vi "Check_EnFlo_Arm.vi"() -> ()   [LabVIEW 2010]
uses:
  Gen Trav/Trav_mode.ctl
  ADAM Serial/Instrument drivers/Traverses/~subVIs/DriveConfigGlobal.vi
panel:
  out "Position Output XYZ":dbl[](array[numeric]) format="%.2f"
  in  "Mode":T1(ring)
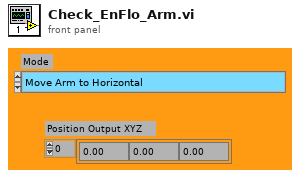
[diagram p1: front panel]
types:
  T1 = enum16{"Move Arm to Horizontal", "Teach Traverse That Arm is Level"}
  T2 = typedef "Trav_mode.ctl" = enum16{"Move traverse", "Read traverse position", "Teach Position"}
  T3 = enum16{"Load setup from excel file", "Save setup to excel file"}
  T4 = typedef "AxisConfigCluster.ctl" = cluster{"Channel Properties":T5, "Static Drive Configuration":T6}
  T5 = typedef "DriveProperties.ctl" = cluster{"Channel Name":string, "Vel. Default":dbl, "Acc. Default":dbl, "Vel. Max":dbl, "Vel. Min":dbl, "Acc. Max":dbl, "Acc. Min":dbl, "Pulses/unit":dbl, "Address":u8, "Pulse Offset":i32, "Pos Tolerance":dbl, "Pulses/rev":dbl, "Backlash/Eng units":dbl, "Current Pos":dbl, "Ch Status":enum16{"Active", "Offline", "Simulate"}, "Port Name":string, "Axis Transform mode":string, "Metadata Ch Name":string, "Type":string}
  T6 = typedef "DriveStaticConfig.ctl" = cluster{"Correction Gain % (CG)":u16, "Dead Band (DB)":i32, "Dead Band Window (DW)":i32, "Encoder Resolution (ER)":i32, "Step Mode  (FSB)":u16, "Position Maintenance (FSC)":u16, "Stop on Stall (FSD)":u16, "Activate OP1 on stall (FSE)":u16, "Stop on Trigger 3 (FSF)":u16, "OP2 in Deadband (FSG)":u16, "Stall Detect (FSH)":u16, "Limit Disable (LD)":u16, "Motor Resolution (MR)":enum16{"200", "400", "1000", "2000", "4000", "5000", "10000", "12800", "18000", "20000", "21600", "25000", "25400", "25600", "36000", "50000", "278528", "425984", "507904", "614400", "655360", "819200", "1024000"}, "Limit Switch Sense (OSA)":u16, "Home Position (OSB)":u16, "Home Switch Sense (OSC)":u16, "Encoder Z for Home (OSD)":u16, "Reference edge of Home (OSH)":u16, "RS232 Echo Control (SSA)":u16, "Buffer at Limit (SSG)":u16, "Buffer at Stop (SSH)":u16, "Indexer Mode  (FSA)":u16, "Type":string, "ConfigString":string, "De Power Motor":enum16{"TRUE", "FALSE"}}
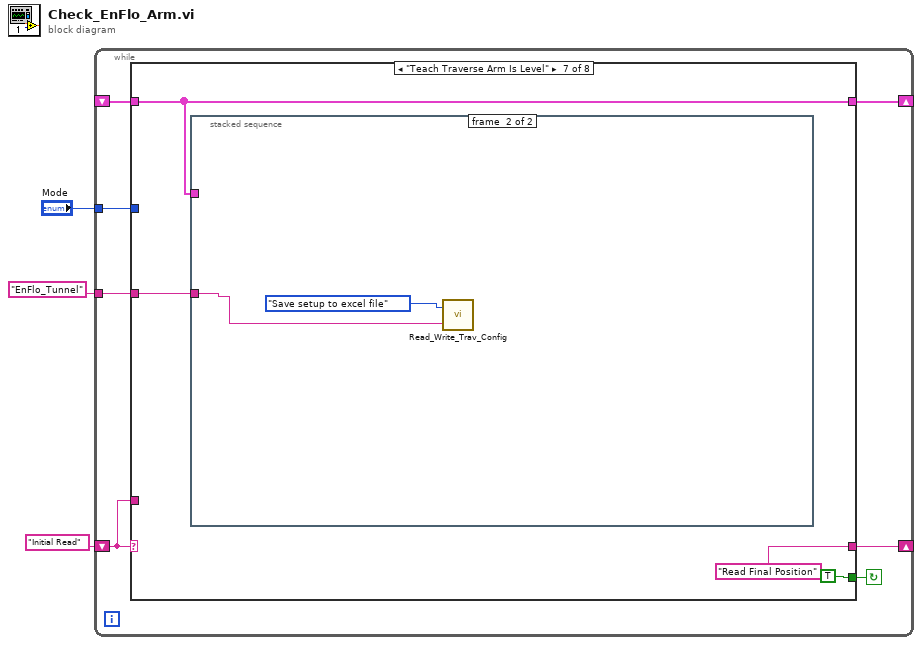
[diagram p0: block diagram]
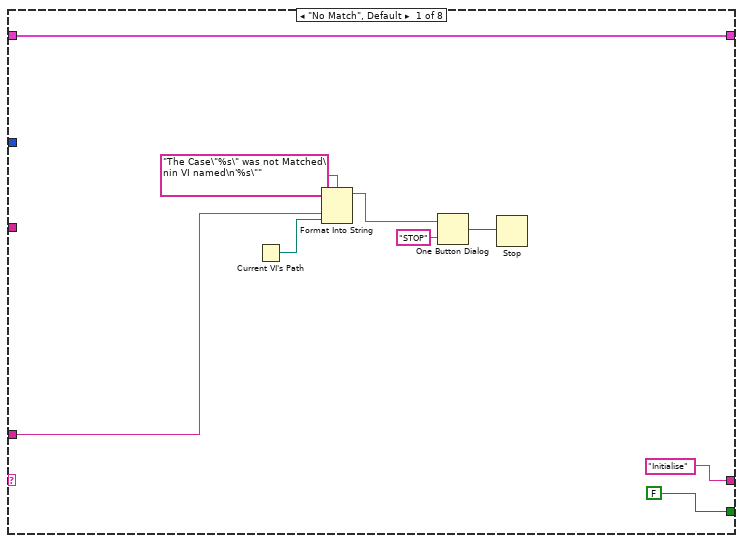
[diagram p2: hidden frame]
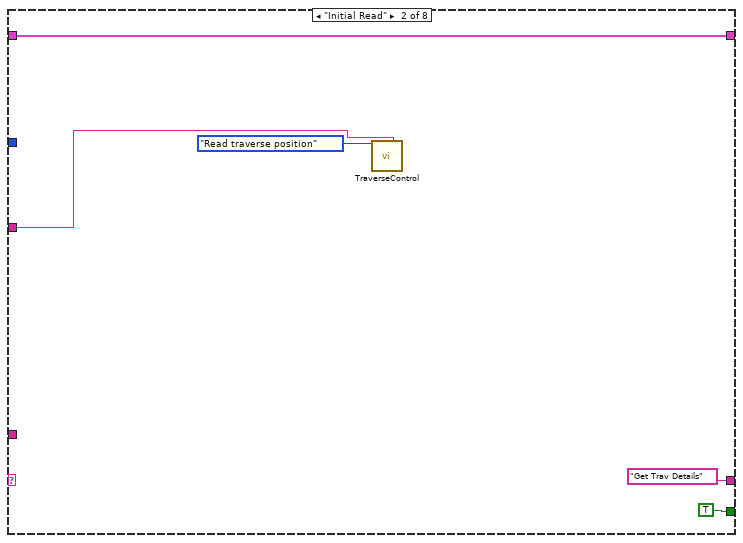
[diagram p3: hidden frame]
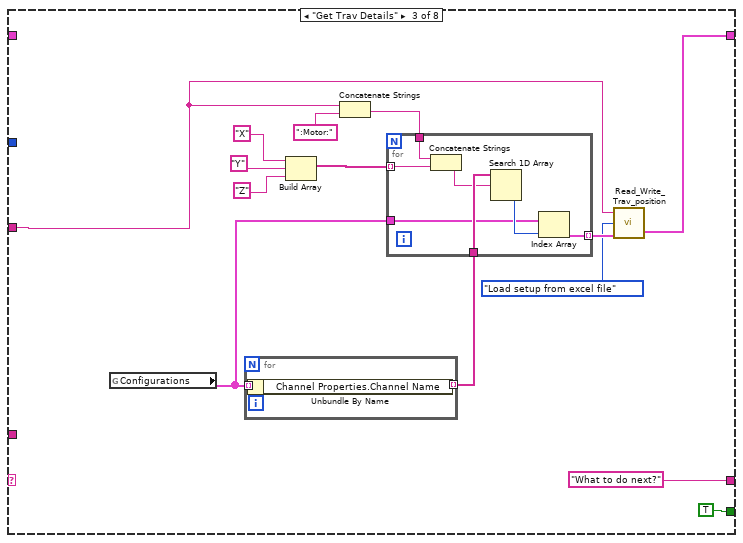
[diagram p4: hidden frame]
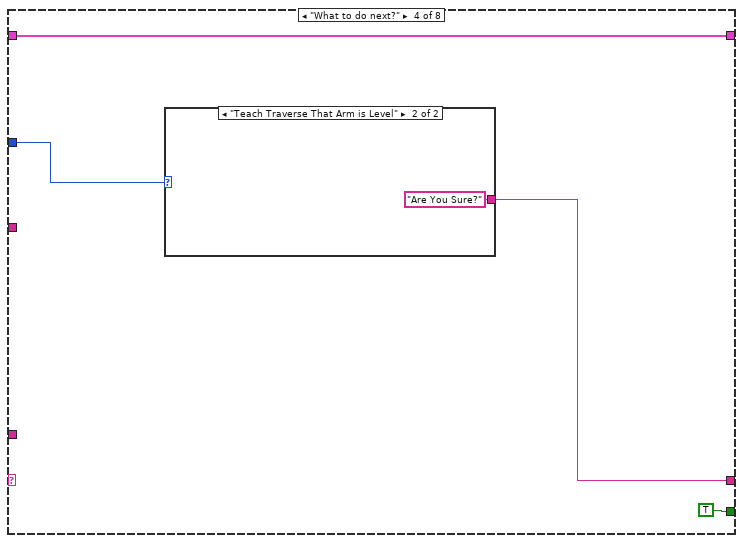
[diagram p5: hidden frame]
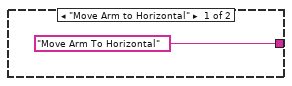
[diagram p6: hidden frame]
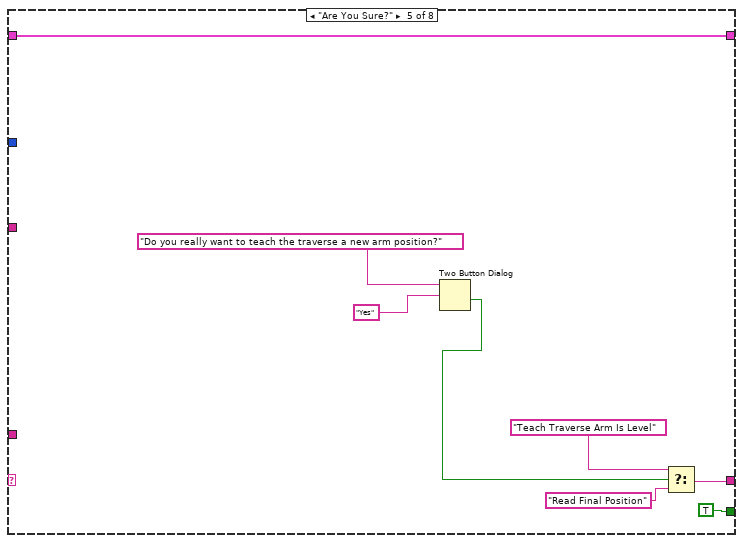
[diagram p7: hidden frame]
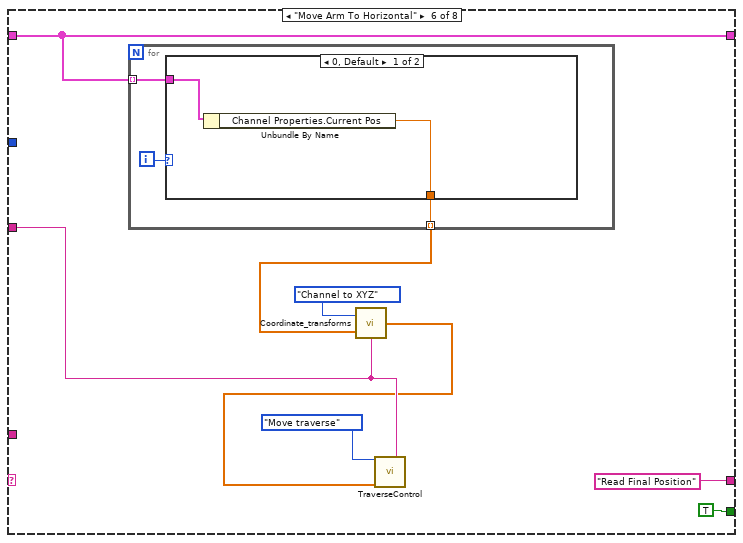
[diagram p8: hidden frame]
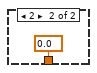
[diagram p9: hidden frame]
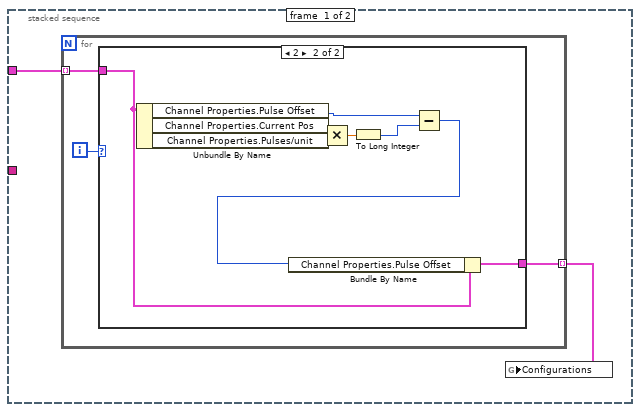
[diagram p10: hidden frame]
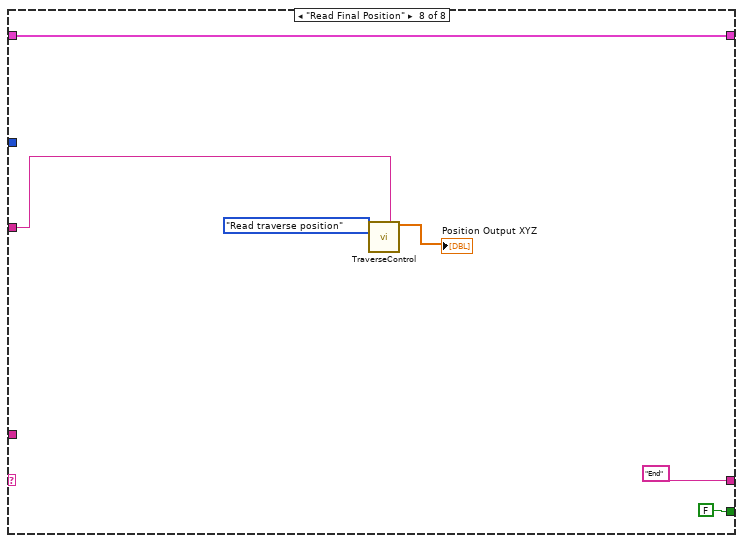
[diagram p12: hidden frame]
diagram:
  n1 = while {
    tunnel: "Mode" -> [w4]
    shift-left: _ -> [w5]
    shift-right: [w6] -> _
    tunnel: "EnFlo_Tunnel" ("Traverse Name") -> [w7]
    shift-left: "Initial Read" -> [w8]
    shift-right: [w9] -> _
    stop <- w10 continue-if-true
    n2 = case shown="\"Teach Traverse Arm Is Level\"" w8 {
      tunnel: [FALSE TRUE TRUE TRUE TRUE TRUE TRUE FALSE] -> w10
      tunnel: ["Initialise" "Get Trav Details" "What to do next?" w49 w55 "Read Final Position" "Read Final Position" "End"] -> w9
      tunnel: w8 -> [w14 _ _ _ _ _ _ _]
      tunnel: w7 -> [_ w20 w26 _ _ w64 w76 w98]
      tunnel: [w11 w21 w25 w48 w60 w67 w77 w97] -> w6
      tunnel: w5 -> [w11 w21 _ w48 w60 w67 w77 w97]
      tunnel: w4 -> [_ _ _ w50 _ _ _ _]
      frame "No Match", Default {
        n3 = Current VI's Path() -> (path=w13:path)
        n4 = Format Into String(format string="The Case\"%s\" was not Matched\nin VI named\n'%s\"" ("Format String"), w14, w13) -> (resulting string=w17:string)  [unwired: 2 in, 1 out]
        n5 = One Button Dialog(message=w17, button name ("OK")="STOP") -> (true=w15:bool)
        n6 = Stop(stop? (T)=w15) -> ()
      }
      frame "Initial Read" {
        n7 = call "TraverseControl.vi"("Mode"=Trav_mode."Read traverse position", "Traverse Name"=w20) -> ()  [unwired: 12 in, 2 out]
      }
      frame "Get Trav Details" {
        n8 = global read "DriveConfigGlobal.vi" "Configurations"() -> (w29:T4[])
        n9 = for {
          tunnel: w29 -> [w40] mode=indexing
          tunnel: [w39] -> w30 mode=indexing
          n10 = Unbundle By Name(w40) -> ("Channel Properties.Channel Name"=w39:string)
        }
        n11 = Build Array("X", "Y", "Z") -> (w35:string[])
        n12 = Concatenate Strings(w26, ":Motor:") -> (w34:string)
        n13 = for {
          tunnel: w35 -> [w47] mode=indexing
          tunnel: w34 -> [w46]
          tunnel: w30 -> [w45]
          tunnel: w29 -> [w42]
          tunnel: [w41] -> w28 mode=indexing
          n14 = Concatenate Strings(w46, w47) -> (w44:string)
          n15 = Search 1D Array(1D array=w45, element=w44) -> (index of element=w43:i32)  [unwired: 1 in]
          n16 = Index Array(array=w42, index=w43) -> (element=w41:T4)
        }
        n17 = call "Read_Write_Trav_position.vi"("Matched Configurations In"=w28, "Mode"=T3."Load setup from excel file", "Traverse Name"=w26) -> ("Matched Configurations Out"=w25:T4[])  [unwired: 1 in]
      }
      frame "What to do next?" {
        n18 = case shown="\"Teach Traverse That Arm is Level\"" w50 {
          tunnel: ["Move Arm To Horizontal" "Are You Sure?"] -> w49
          frame "Move Arm to Horizontal" {
          }
          frame "Teach Traverse That Arm is Level" {
          }
        }
      }
      frame "Are You Sure?" {
        n19 = Two Button Dialog(message="Do you really want to teach the traverse a new arm position?", 2:"Yes" ("T button name (\"OK\")")) -> (T button?=w57:bool)  [unwired: 1 in]
        n20 = Select(t="Teach Traverse Arm Is Level", s=w57, f="Read Final Position") -> (s? t:f=w55:string)
      }
      frame "Move Arm To Horizontal" {
        n21 = for {
          tunnel: w67 -> [w71] mode=indexing
          tunnel: [w70] -> w65 mode=indexing
          i -> [w72]
          n22 = case shown="0, Default" w72 {
            tunnel: w71 -> [w74 _]
            tunnel: [w73 0.0 ("Current Pos")] -> w70
            frame 0, Default {
              n23 = Unbundle By Name(w74) -> ("Channel Properties.Current Pos"=w73:dbl)
            }
            frame 2 {
            }
          }
        }
        n24 = call "Coordinate_transforms.vi"("Traverse Name"=w64, "Input"=w65, "Mode"=enum16{"XYZ to Channel", "Channel to XYZ"}."Channel to XYZ") -> ("Output"=w63:dbl[])
        n25 = call "TraverseControl.vi"("Mode"=Trav_mode."Move traverse", "Traverse Name"=w64, "Position input XYZ"=w63) -> ()  [unwired: 11 in, 2 out]
      }
      frame "Teach Traverse Arm Is Level" {
        n26 = stacked-sequence {
          tunnel: w77 -> [w81 _]
          tunnel: w76 -> [_ w94]
          frame #0 {
            n27 = for {
              tunnel: w81 -> [w83] mode=indexing
              tunnel: [w82] -> w80 mode=indexing
              i -> [w84]
              n28 = case shown="2" w84 {
                tunnel: w83 -> [w85 w90]
                tunnel: [w85 w86] -> w82
                frame 0, Default {
                }
                frame 2 {
                  n29 = Unbundle By Name(w90) -> ("Channel Properties.Pulse Offset"=w91:i32, "Channel Properties.Current Pos"=w93:dbl, "Channel Properties.Pulses/unit"=w92:dbl)
                  n30 = Multiply(x=w93, y=w92) -> (x*y=w89:dbl)
                  n31 = To Long Integer(number=w89) -> (32bit integer=w88:i32)
                  n32 = Subtract(x=w91, y=w88) -> (x-y=w87:i32)
                  n33 = Bundle By Name(cluster=w90, "Channel Properties.Pulse Offset"=w87) -> (w86:T4)
                }
              }
            }
            n34 = global write "DriveConfigGlobal.vi" "Configurations"(w80) -> ()
          }
          frame #1 {
            n35 = call "Read_Write_Trav_Config.vi"("Traverse Name"=w94, "Mode"=T3."Save setup to excel file") -> ()  [unwired: 1 in]
          }
        }
      }
      frame "Read Final Position" {
        n36 = call "TraverseControl.vi"("Mode"=Trav_mode."Read traverse position", "Traverse Name"=w98) -> ("Position Output XYZ"=→"Position Output XYZ":dbl[])  [unwired: 12 in, 1 out]
      }
    }
  }
